vi "Acquire.vi"(8 "error in (no error)":errorcluster, 9 "Min Value":dbl, 10 "Max Value":dbl, 11 "Refnum in":refnum<k21>) -> (0 "error out":errorcluster, 2 "Graph Data":waveform(dbl)[](array[waveform]))   [LabVIEW 2019, in "Acquisition.lvlib"]
doc: "Perform the acquisition. Replace the contents of this diagram with calls to acquisition hardware.\n_____\nBased on Delacor QMH Project Template 5.0.0.82."
uses:
  Acquisition.lvlib
  <vilib>/ULx/Create Channel.llb/ULx Create Channel (AI-Voltage-Basic).vi
  <vilib>/ULx/Timing.llb/ULx Timing (Sample Clock).vi
  <vilib>/ULx/Read.llb/ULx Read (Analog Wfm 1Chan NSamp).vi
  <vilib>/express/express shared/ex_Modify Signal Name.vi
  <vilib>/express/express arith-compare/Formula/XNode/ExpressFormulaBlockNode.xnode
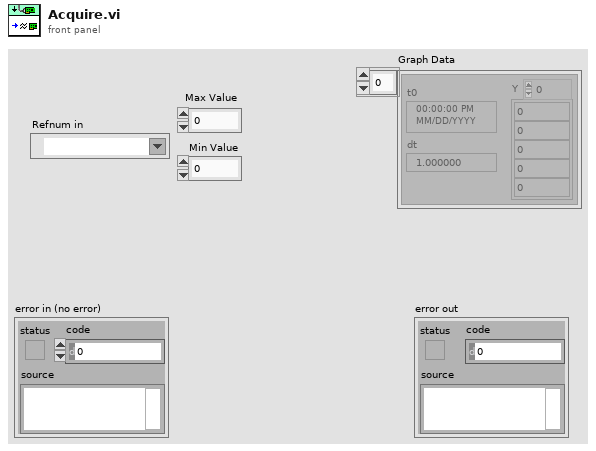
[diagram p1: front panel]
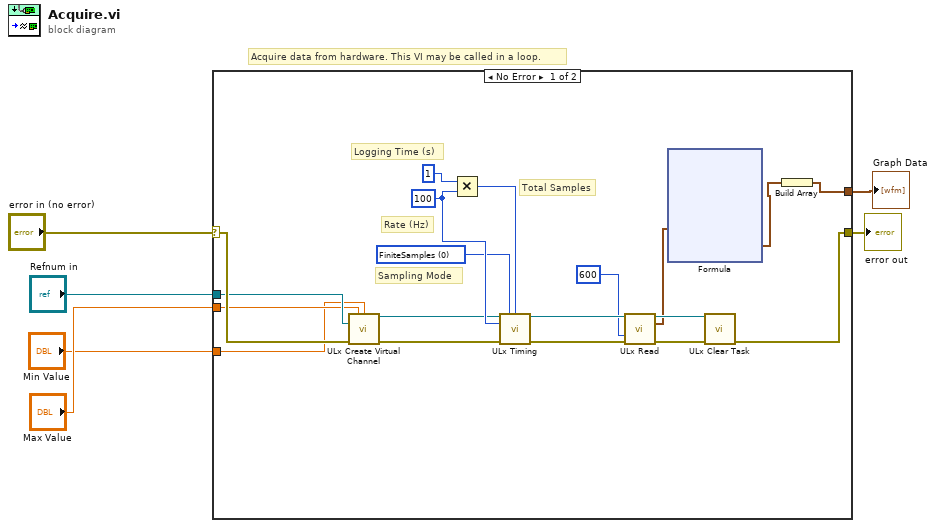
[diagram p0: block diagram]
diagram:
  # "Acquire data from hardware. This VI may be called in a loop."
  n1 = case shown="No Error" "error in (no error)" {
    selector: "error in (no error)" -> [w13 w40]
    tunnel: [w14 w40] -> w5
    tunnel: [w7 _] -> w4
    tunnel: "Refnum in" -> [w12 _]
    tunnel: "Max Value" -> [w11 _]
    tunnel: "Min Value" -> [w10 _]
    frame No Error {
      w16 = 0 items=["FiniteSamples", "ContinuousSamples"] ("Sampling Mode")
      w21 = 100
      # "Sampling Mode"
      # "Total Samples"
      # "Logging Time (s)"
      # "Rate (Hz)"
      n2 = call-poly <vilib>:"ULx Create Virtual Channel.vi"("maximum value"=w11, "minimum value"=w10, "physical channels"=w12, "error in"=w13) -> ("task out"=w20:refnum<k24>, "error out"=w24:errorcluster)  [unwired: 10 in]
      n3 = Multiply(x=1, y=w21) -> (x*y=w22:i32)
      n4 = call-poly <vilib>:"ULx Timing.vi"("task in"=w20, "sample mode"=w16, "samples per channel"=w22, "rate"=w21, "error in"=w24) -> ("task out"=w19:refnum<k24>, "error out"=w25:errorcluster)  [unwired: 9 in]
      n5 = call-poly <vilib>:"ULx Read.vi"("task in"=w19, "timeout"=600, "error in"=w25) -> ("task out"=w18:refnum<k24>, "data"=w9:waveform(dbl), "error out"=w17:errorcluster)  [unwired: 10 in]
      n6 = xnode "Formula"("X1"=w9) -> ("Result"=w8:waveform(dbl))  [unwired: 1 in, 1 out]
      n7 = call <vilib>:"ULx Clear Task.vi"("task in"=w18, "error in"=w17) -> ("error out"=w14:errorcluster)  [unwired: 13 in]
      n8 = Build Array(w8) -> (w7:waveform(dbl)[])
    }
    frame Error {
    }
  }
  "error out" <- w5
  "Graph Data" <- w4
